vi "Create Default Attributes.vi"(5 "Unique ID":string, 7 "Process Executive Ref":refnum<data-value>, 11 "Start Spot Free Rinse in":refnum<class "Start Spot Free Rinse.lvclass">) -> (3 "Start Spot Free Rinse out":refnum<class "Start Spot Free Rinse.lvclass">)   [LabVIEW 2019, in "Start Spot Free Rinse.lvclass"]
uses:
  <vilib>/gpm_packages/@cs/Car-wash/Source/Process Steps/Start Spot Free Rinse/Start Spot Free Rinse.lvclass
  <vilib>/gpm_packages/@cs/test-executive/Source/Test Executive/ITestExecutive/ITest Executive.lvclass
  94979c9f-0512-495b-b42d-c4c7d8642097.vi
  <vilib>/Utility/error.llb/Error Cluster From Error Code.vi
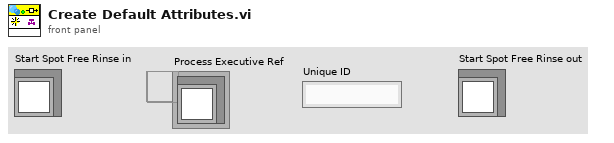
[diagram p1: front panel]
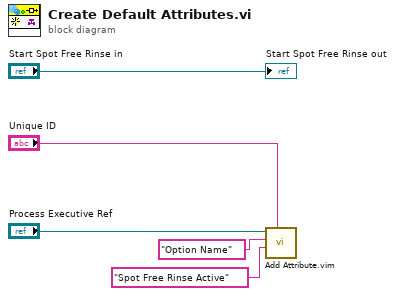
[diagram p0: block diagram]
diagram:
  n1 = call "Add Attribute.vim"("ID"="Unique ID", "Attribute"="Spot Free Rinse Active" ("Item Name"), "Attribute Name"="Option Name" ("Item Name"), "Test Executive Ref"="Process Executive Ref") -> ()  [unwired: 4 in, 4 out]
  "Start Spot Free Rinse out" <- "Start Spot Free Rinse in"
